vi "Try1.vi"() -> ()   [LabVIEW 2011]
uses:
  <vilib>/Utility/file.llb/Read From Spreadsheet File (string).vi
panel:
  out "String":string
  in  "index":i32
  out "element":string
  out "size(s)":i32
  out "first row":string[](array[string])
  in  "file path (dialog if empty)":path
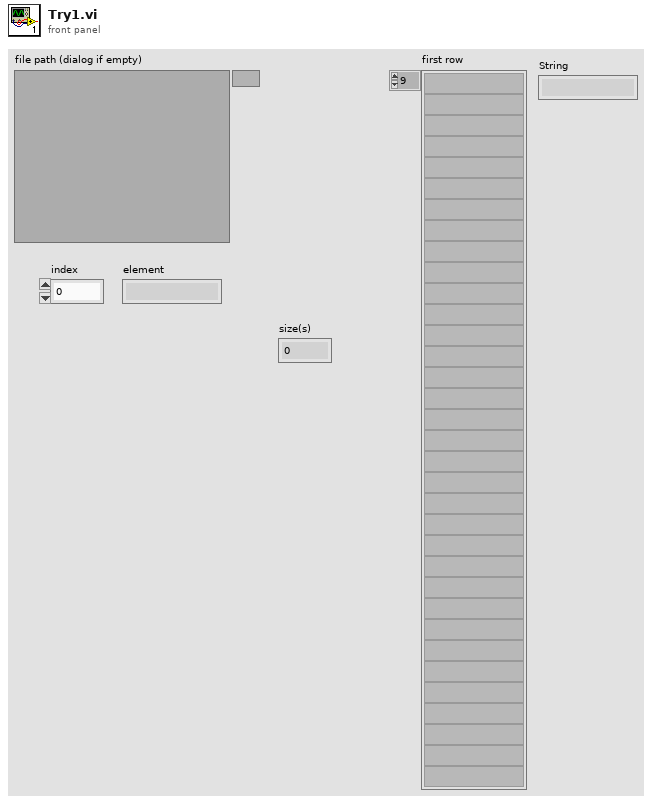
[diagram p1: front panel]
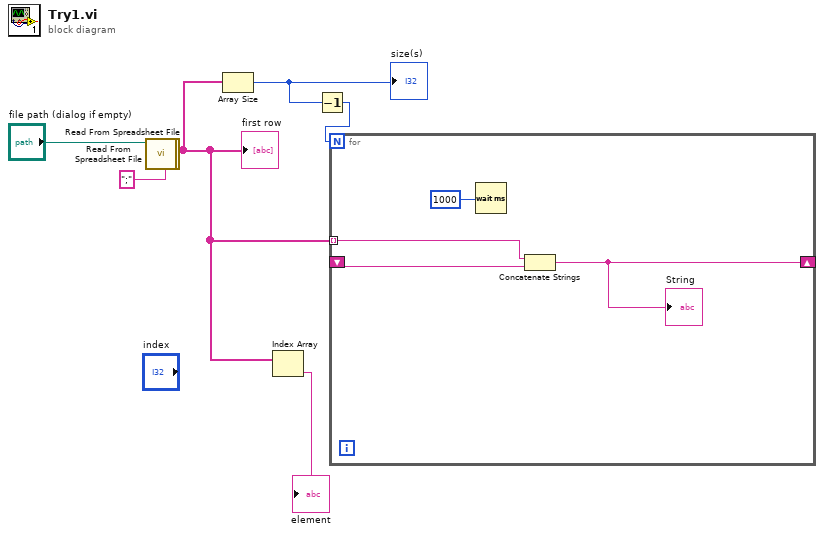
[diagram p0: block diagram]
diagram:
  n1 = call-poly <vilib>:"Read From Spreadsheet File.vi"("delimiter (\\t)"=";" ("delimiter (\\t)"), "file path (dialog if empty)"="file path (dialog if empty)") -> ("first row"=w1:string[])  [unwired: 5 in, 4 out]
  "first row" <- w1
  n2 = call-poly <vilib>:"Read From Spreadsheet File.vi"() -> ()  [unwired: 7 in, 5 out]
  n3 = Array Size(array=w1) -> (size(s)=w3:i32)
  "size(s)" <- w3
  n4 = Index Array(array=w1) -> (element=→"element":string)  [unwired: 1 in]
  n5 = Decrement(x=w3) -> (x-1=w4:i32)
  n6 = for {
    N: w4 -> [_]
    tunnel: w1 -> [w9] mode=indexing
    shift-right: [w7] -> _
    shift-left: _ -> [w8]
    n7 = Wait (ms)(milliseconds to wait=u32 1000 ("millisecond timer value")) -> ()  [unwired: 1 out]
    n8 = Concatenate Strings(w9, w8) -> (w7:string)
    "String" <- w7
  }
